vi "DO-NOT-USE_setDelay.vi"(8 "error in (no error)":errorcluster, 9 "Rate (ps/s)":dbl, 10 "Delay (ps)":dbl, 11 "Instrument.Delay in":refnum<class "Instrument.Aerotech.lvclass">) -> (0 "error out":errorcluster, 3 "Instrument.Delay out":refnum<class "Instrument.Aerotech.lvclass">)   [LabVIEW 2019, in "Instrument.Aerotech.lvclass"]
uses:
  Instrument.Aerotech.lvclass
  Instrument.Aerotech.lvclass/Instrument.Aerotech.ctl
  Aerotech-Ensemble-LabVIEW/2010-5.6/Motion/MoveAbsSingle.vi
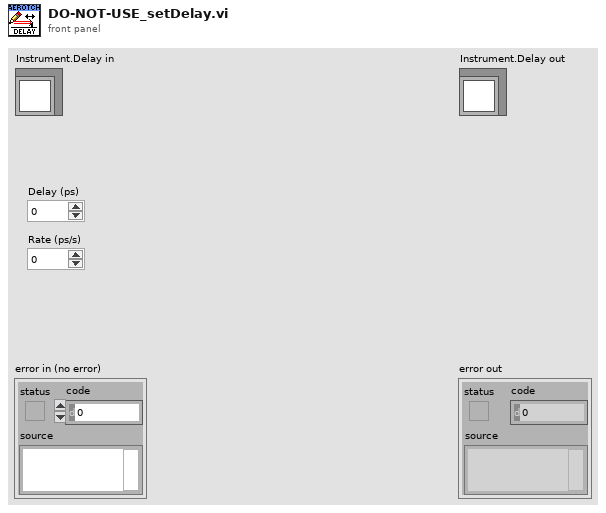
[diagram p1: front panel]
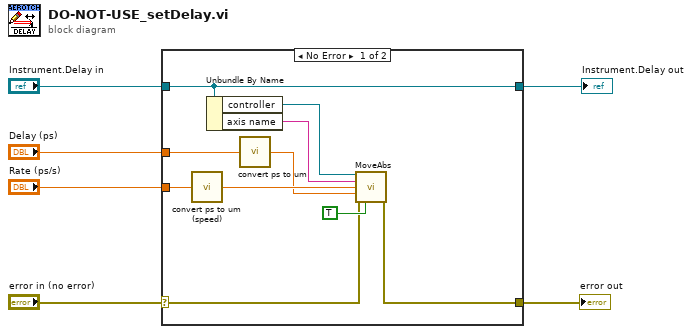
[diagram p0: block diagram]
diagram:
  n1 = case shown="No Error" "error in (no error)" {
    selector: "error in (no error)" -> [w13 w18]
    tunnel: [w7 w18] -> w6
    tunnel: "Delay (ps)" -> [w11 _]
    tunnel: "Rate (ps/s)" -> [w10 _]
    tunnel: "Instrument.Delay in" -> [w12 w17]
    tunnel: [w12 w17] -> w1
    frame No Error {
      n2 = call "convert ps to um (speed).vi"("Delay speed (ps/s)"=w10) -> ("Position speed (um/s)"=w9:dbl)
      n3 = Unbundle By Name(w12) -> ("controller"=w15:refnum<k24>, "axis name"=w14:string)
      n4 = call "convert ps to um.vi"("Delay (ps)"=w11) -> ("Position (um)"=w8:dbl)
      n5 = call-poly "MoveAbs.vi"("controller in"=w15, "axis name"=w14, "speed"=w9, "distance"=w8, "error in (no error)"=w13, "return immediately"=TRUE) -> ("error out"=w7:errorcluster)  [unwired: 8 in, 1 out]
    }
    frame Error {
    }
  }
  "error out" <- w6
  "Instrument.Delay out" <- w1
